vi "Draw TextBox.vi"(7 "attitude (rad)":T1, 9 "draw options":T2={"Text Color"=16777238, "Wing Color"=16751616, "Dial Outline Color"=13816530, "Sky Color"=3381759, "Ground Color"=8213043, "Horizon Line Color"=16777225, "Outline Color"=0, "Dial Background Color"=5987163, "Draw Wings"=TRUE, "Draw Text"=TRUE, "Font Name"="Helvetica", "Angle units"=enum."Degrees"}, 10 "draw area state":T4, 11 "picture in":picture) -> (3 "picture out":picture)   [LabVIEW 2017, in "NI_Robotics_Attitude Picture.lvlib"]
uses:
  <vilib>/robotics/Controls/Attitude Indicator/Attitude Picture/NI_Robotics_Attitude Picture.lvlib
  <vilib>/robotics/Controls/Attitude Indicator/Attitude Picture/Draw Area State.ctl
  <vilib>/Utility/miscctls.llb/LVBoundsTypeDef.ctl
  <vilib>/robotics/Controls/Attitude Indicator/Attitude Picture/Draw Options.ctl
  <vilib>/robotics/Controls/Utilities/Angle Units.ctl
  <vilib>/robotics/Controls/Attitude Indicator/Attitude Picture/Attitude.ctl
  <vilib>/Analysis/coordinate.llb/2D Cartesian Coordinate Rotation.vi
  <vilib>/Analysis/coordinate.llb/2D Cartesian Coordinate Rotation (Array).vi
  <vilib>/picture/picture.llb/Get Text Rect.vi
  <vilib>/Utility/AngleManip/Radians to Degrees.vi
  <vilib>/Utility/AngleManip/Radians to Degrees (Scalar DBL).vi
  <vilib>/robotics/Controls/Utilities/NI_Robotics_Control Utilities.lvlib
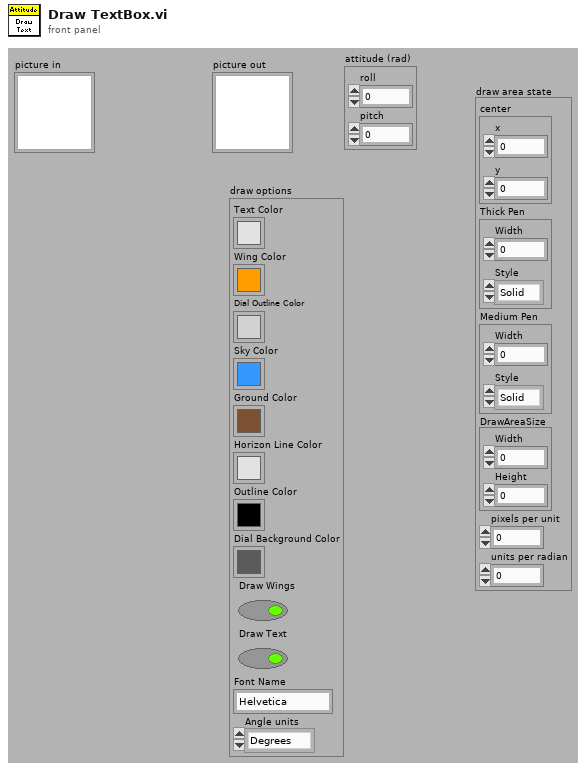
[diagram p1: front panel]
types:
  T1 = typedef "NI_Robotics_Attitude Picture.lvlib/Attitude.ctl" = cluster{"roll":dbl, "pitch":dbl}
  T2 = typedef "NI_Robotics_Attitude Picture.lvlib/Draw Options.ctl" = cluster{"Text Color":u32, "Wing Color":u32, "Dial Outline Color":u32, "Sky Color":u32, "Ground Color":u32, "Horizon Line Color":u32, "Outline Color":u32, "Dial Background Color":u32, "Draw Wings":bool, "Draw Text":bool, "Font Name":string, "Angle units":T3}
  T3 = typedef "NI_Robotics_Control Utilities.lvlib/Angle Units.ctl" = enum16{"Radians", "Degrees"}
  T4 = typedef "NI_Robotics_Attitude Picture.lvlib/Draw Area State.ctl" = cluster{"center":cluster{"x":i16, "y":i16}, "Thick Pen":cluster{"Width":u16, "Style":enum32{"Solid", "Dash", "Dot", "DashDot", "DashDotDot"}}, "Medium Pen":cluster{"Width":u16, "Style":enum32{"Solid", "Dash", "Dot", "DashDot", "DashDotDot"}}, "DrawAreaSize":T5, "pixels per unit":dbl, "units per radian":dbl}
  T5 = typedef "LVBoundsTypeDef.ctl" = cluster{"Width":u32, "Height":u32}
  T6 = cluster{"left":i16, "top":i16, "right":i16, "bottom":i16}
  T7 = cluster{"Width":i16, "Style":enum32{"Solid", "Dash", "Dot", "DashDot", "DashDotDot"}}
  T8 = cluster{"horizontal":enum16{"left", "center", "right"}, "vertical":enum16{"top", "center", "bottom"}}
  T9 = enum16{"User-specified Font", "Application Font", "System Font", "Dialog Font"}
  T10 = cluster{"Font Name:":string, "Size":i16, "Strikeout?":bool, "Italic?":bool, "Underline?":bool, "Outline?":bool, "Shadow?":bool, "Bold?":bool}
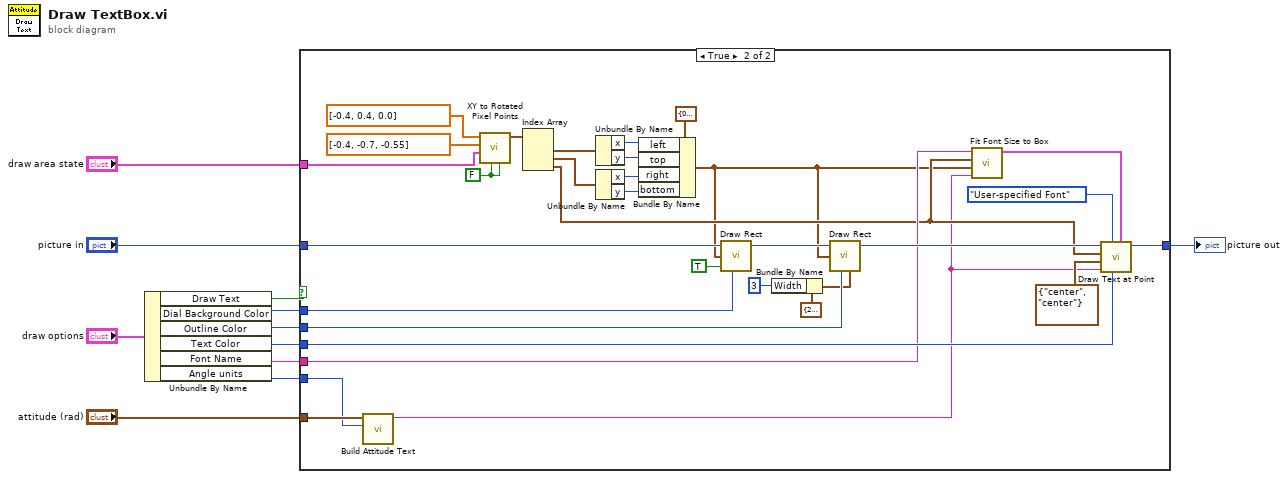
[diagram p0: block diagram]
diagram:
  n1 = Unbundle By Name("draw options") -> ("Draw Text"=w1:bool, "Dial Background Color"=w7:u32, "Outline Color"=w6:u32, "Text Color"=w5:u32, "Font Name"=w4:string, "Angle units"=w2:T3)
  n2 = case shown="True" w1 {
    tunnel: [w12 w44] -> w11
    tunnel: "picture in" -> [w12 w20]
    tunnel: "draw area state" -> [_ w32]
    tunnel: w7 -> [_ w40]
    tunnel: w6 -> [_ w39]
    tunnel: w5 -> [_ w38]
    tunnel: w4 -> [_ w17]
    tunnel: "attitude (rad)" -> [_ w37]
    tunnel: w2 -> [_ w36]
    frame False {
    }
    frame True {
      w35 = FALSE ("use pitch")
      n3 = call <vilib>:"Build Attitude Text.vi"("angle units"=w36, "attitude (rad)"=w37) -> ("text"=w13:string)  [unwired: 9 in]
      n4 = call <vilib>:"XY to Rotated Pixel Points.vi"("use roll"=w35, "use pitch"=w35, "draw area state"=w32, "unrotated y (units)"=dbl[] [-0.4, -0.7, -0.55] ("unrotated x (units)"), "unrotated x (units)"=dbl[] [-0.4, 0.4, 0.0]) -> ("rotated pixel points"=w31:cluster{"x":i16, "y":i16}[])  [unwired: 6 in]
      n5 = Index Array(array=w31) -> (element #1=w29:cluster{"x":i16, "y":i16}, element #2=w26:cluster{"x":i16, "y":i16}, element #3=w15:cluster{"x":i16, "y":i16})  [unwired: 3 in]
      n6 = Unbundle By Name(w29) -> ("x"=w28:i16, "y"=w27:i16)
      n7 = Unbundle By Name(w26) -> ("x"=w25:i16, "y"=w24:i16)
      n8 = Bundle By Name(cluster=T6 {"left"=0, "top"=0, "right"=0, "bottom"=0} ("rect"), "left"=w28, "top"=w27, "right"=w25, "bottom"=w24) -> (w14:T6)
      n9 = call <vilib>:"Draw Rect.vi"("picture"=w20, "rect"=w14, "fill?(F)"=TRUE, "color(black)"=w40) -> ("new picture"=w19:picture)  [unwired: 5 in]
      n10 = Bundle By Name(cluster=T7 {"Width"=2, "Style"=enum."Solid"} ("pen"), "Width"=i16 3) -> (w22:T7)
      n11 = call <vilib>:"Draw Rect.vi"("picture"=w19, "rect"=w14, "color(black)"=w39, "pen"=w22) -> ("new picture"=w18:picture)  [unwired: 5 in]
      n12 = call <vilib>:"Fit Font Size to Box.vi"("text"=w13, "box rect"=w14, "box center"=w15, "font name"=w17) -> ("font"=w16:T10)  [unwired: 7 in]
      n13 = call <vilib>:"Draw Text at Point.vi"("[user-specified font]"=w16, "text color(black)"=w38, "desired font(Application)"=T9."User-specified Font", "text"=w13, "alignment(left, top)"=T8 {"horizontal"=enum."center", "vertical"=enum."center"}, "origin"=w15, "picture"=w18) -> ("new picture"=w44:picture)  [unwired: 3 in, 1 out]
    }
  }
  "picture out" <- w11
